vi "Send Go  POS.vi"(5 "Type CMD":string="GoToPos All", 6 "Parameter Data":variant, 7 "XYZ notifier":refnum<notifier>, 8 "error in (no error)":errorcluster, 11 "Motor Queue in":refnum<queue>) -> (0 "error out":errorcluster, 2 "timed out?":bool)   [LabVIEW 2020]
uses:
  support/Message Queue/Message Cluster.ctl
  support/Message Queue/Message Queue.lvlib
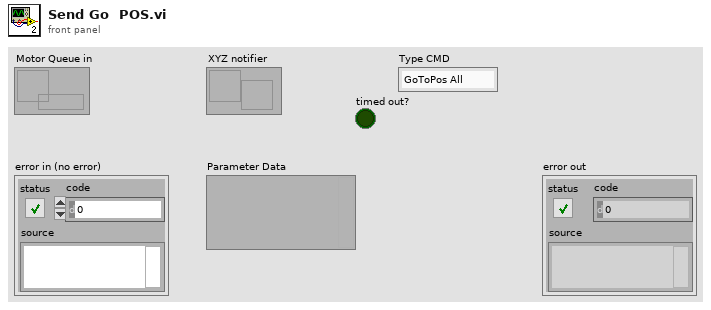
[diagram p1: front panel]
types:
  T1 = cluster{"Type CMD":string, "Mode CMD":string, "Main CMD":string}
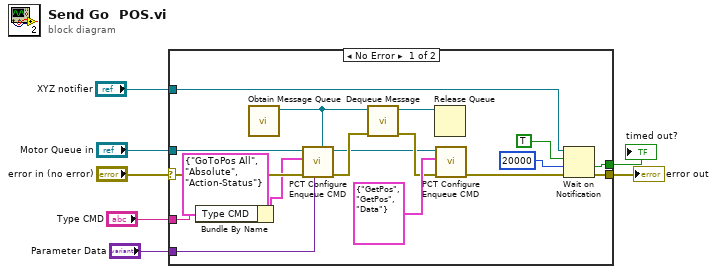
[diagram p0: block diagram]
diagram:
  n1 = case shown="No Error" "error in (no error)" {
    selector: "error in (no error)" -> [w13 w26]
    tunnel: "XYZ notifier" -> [w15 _]
    tunnel: "Motor Queue in" -> [w14 _]
    tunnel: [w12 w26] -> w4
    tunnel: "Parameter Data" -> [w11 _]
    tunnel: "Type CMD" -> [w9 _]
    tunnel: [w8 _] -> w1
    frame No Error {
      n2 = Bundle By Name(cluster=T1 {"Type CMD"="GoToPos All", "Mode CMD"="Absolute", "Main CMD"="Action-Status"} ("CMD"), "Type CMD"=w9) -> (w10:T1)
      n3 = call "Obtain Message Queue.vi"() -> ("Message Queue"=w19:refnum<queue>)  [unwired: 10 in, 1 out]
      n4 = call "PCT Configure Enqueue CMD.vi"("Response Queue"=w19, "Parameter Data"=w11, "error in (no error)"=w13, "CMD"=w10, "CMD Queue in"=w14) -> ("error out"=w20:errorcluster, "CMD Queue out"=w16:refnum<queue>)  [unwired: 4 in, 1 out]
      n5 = call "Dequeue Message.vi"("error in (no error)"=w20, "Message Queue"=w19) -> ("error out"=w17:errorcluster, "dup Message Queue"=w18:refnum<queue>)  [unwired: 6 in, 2 out]
      n6 = Release Queue(queue=w18) -> ()  [unwired: 2 in, 3 out]
      n7 = call "PCT Configure Enqueue CMD.vi"("error in (no error)"=w17, "CMD"=T1 {"Type CMD"="GetPos", "Mode CMD"="GetPos", "Main CMD"="Data"}, "CMD Queue in"=w16) -> ("error out"=w23:errorcluster)  [unwired: 6 in, 2 out]
      n8 = Wait on Notification(notifier=w15, ignore previous (F)=TRUE, timeout in ms (-1)=20000, error in (no error)=w23) -> (timed out?=w8:bool, error out=w12:errorcluster)  [unwired: 2 out]
    }
    frame Error {
    }
  }
  "error out" <- w4
  "timed out?" <- w1
